vi "Time Left.vi"(9 "Time Elapsed\nper slow":dbl, 10 "Current slow pos":dbl, 11 "Slow array size":dbl) -> (2 "Estimated Time \nLeft":dbl, 3 "Percent Complete":dbl)   [LabVIEW 2021]
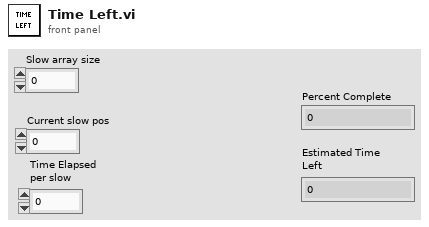
[diagram p1: front panel]
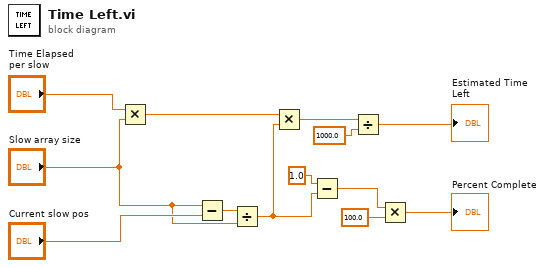
[diagram p0: block diagram]
diagram:
  n1 = Multiply(x="Time Elapsed\nper slow", y="Slow array size") -> (x*y=w2:dbl)
  n2 = Subtract(x="Slow array size", y="Current slow pos") -> (x-y=w12:dbl)
  n3 = Divide(x=w12, y="Slow array size") -> (x/y=w10:dbl)
  n4 = Multiply(x=w2, y=w10) -> (x*y=w6:dbl)
  n5 = Subtract(x=1.0, y=w10) -> (x-y=w8:dbl)
  n6 = Divide(x=w6, y=1000.0) -> (x/y=→"Estimated Time \nLeft":dbl)
  n7 = Multiply(x=w8, y=100.0) -> (x*y=→"Percent Complete":dbl)
